vi "DFD Build MRate Filter from TF (Rational).vi"(6 "fs in [Hz]":dbl=1.0 format="%#_2g", 8 "error in (no error)":errorcluster, 10 "factor":T1, 11 "h(n)":dbl[](array[numeric])) -> (0 "error out":errorcluster, 3 "multirate filter out":T2={"mMRate_Structure"=enum."IIR", "mMRate_Mode"=0, "mMRate_Factor"=-1, "mMRate_FIRParams"={"mMRate_FIR_H"=[], "mMRate_FIR_IsNyquist?"=FALSE, "mMRate_FIR_IsSymmetric?"=FALSE}, "mMRate_CICParams"={"mMRate_CIC_#Stage"=0, "mMRate_CIC_Lag"=0, "mMRate_CIC_Type"=enum."Lowpass"}, "mMRate_Order"=0, "mMRate_Version"="2.0", "mMRate_Comments"="", "mMRate_RationalFactor"={"mMRate_L"=-1, "mMRate_M"=-1}, "mMRate_Fs"=1.0, "mMRate_Quantized?"=FALSE, "mMRate_QFilterGain"=1.0, "mMRate_CoefWl"=16, "mMRate_Scaling"={"mMRate_ScaleByPowerOf2?"=FALSE, "mMRate_ScaleType"=enum."No Norm"}, "mMRate_InputWl"=16, "mMRate_OutputWl"=16, "mMRate_OutputMode"=enum."Truncation", "mMRate_MultMode"=enum."Truncated", "mMRate_BitPruning"=FALSE, "mMRate_GainWl"=16, "mMRate_OutputFwl"=0, "mMRate_SumIwl"=0, "mMRate_InputIwl "=16, "mMRate_SumWl"=32, "mMRate_CoefIwl"=0} {"mMRate_SumWl" min=1 max=32 step=1; "mMRate_InputIwl" min=1 max=32 step=1; "mMRate_GainWl" min=1 max=32 step=1; "mMRate_OutputWl" min=1 max=32 step=1; "mMRate_InputWl" min=1 max=32 step=1; "mMRate_CoefWl" min=1 max=32 step=1; "mMRate_Mode" items=["Default"=-1, "No Rate Change"=0, "Interpolation"=1, "Decimation"=2, "Interpolated"=3, "Rational"=4]})   [LabVIEW 2017, in "NI_DigFilterLicensed.lvlib"]
doc: "Creates a multirate filter. You must manually select the polymorphic instance you want to use."
uses:
  <vilib>/addons/Digital Filter Design/NI_DigFilterLicensed.lvlib
  <vilib>/addons/Digital Filter Design/_Objects.llb/DFD Multirate Filter Obj.ctl
  <vilib>/addons/Digital Filter Design/_Objects.llb/DFD Multirate Mode.ctl
  <vilib>/addons/Digital Filter Design/_Objects.llb/DFD Coef Norm Type.ctl
  <vilib>/addons/Digital Filter Design/_Objects.llb/DFD Round-off Mode.ctl
  <vilib>/addons/Digital Filter Design/_Objects.llb/DFD FXP MRate Multiply Mode.ctl
  <vilib>/addons/Digital Filter Design/_Objects.llb/DFD Multirate Rational Factor.ctl
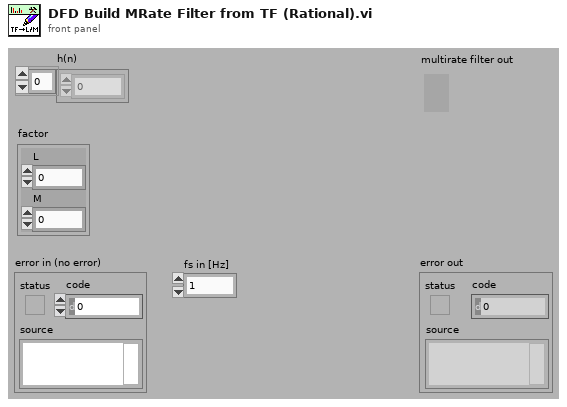
[diagram p1: front panel]
types:
  T1 = typedef "NI_DigFilterLicensed.lvlib/DFD Multirate Rational Factor.ctl" = cluster{"L":i32, "M":i32}
  T2 = typedef "NI_DigFilterLicensed.lvlib/DFD Multirate Filter Obj.ctl" = cluster{"mMRate_Structure":enum16{"CIC", "FIR", "IIR", "Lattice"}, "mMRate_Mode":T3, "mMRate_Factor":i32, "mMRate_FIRParams":cluster{"mMRate_FIR_H":dbl[], "mMRate_FIR_IsNyquist?":bool, "mMRate_FIR_IsSymmetric?":bool}, "mMRate_CICParams":cluster{"mMRate_CIC_#Stage":i32, "mMRate_CIC_Lag":i32, "mMRate_CIC_Type":enum16{"Lowpass", "Highpass"}}, "mMRate_Order":i32, "mMRate_Version":string, "mMRate_Comments":string, "mMRate_RationalFactor":cluster{"mMRate_L":i32, "mMRate_M":i32}, "mMRate_Fs":dbl, "mMRate_Quantized?":bool, "mMRate_QFilterGain":dbl, "mMRate_CoefWl":i16, "mMRate_Scaling":cluster{"mMRate_ScaleByPowerOf2?":bool, "mMRate_ScaleType":T4}, "mMRate_InputWl":i16, "mMRate_OutputWl":i16, "mMRate_OutputMode":T5, "mMRate_MultMode":T6, "mMRate_BitPruning":bool, "mMRate_GainWl":i16, "mMRate_OutputFwl":i16, "mMRate_SumIwl":i16, "mMRate_InputIwl ":i16, "mMRate_SumWl":i16, "mMRate_CoefIwl":i16}
  T3 = typedef "NI_DigFilterLicensed.lvlib/DFD Multirate Mode.ctl" = i16
  T4 = typedef "NI_DigFilterLicensed.lvlib/DFD Coef Norm Type.ctl" = enum16{"No Norm", "Time Domain 1-Norm", "Time Domain 2-Norm", "Time Domain Inf-Norm"}
  T5 = typedef "NI_DigFilterLicensed.lvlib/DFD Round-off Mode.ctl" = enum16{"Nearest", "Truncation"}
  T6 = typedef "NI_DigFilterLicensed.lvlib/DFD FXP MRate Multiply Mode.ctl" = enum16{"Truncated", "Full"}
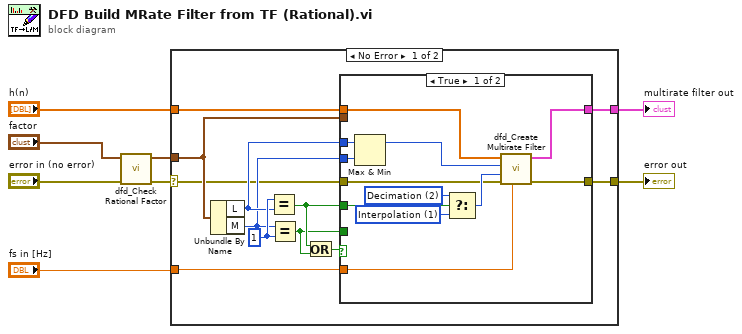
[diagram p0: block diagram]
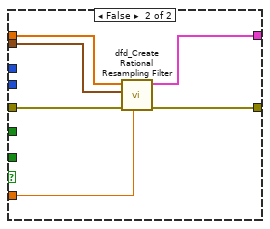
[diagram p2: hidden frame]
diagram:
  n1 = call <vilib>:"dfd_Check Rational Factor.vi"("error in (no error)"="error in (no error)", "rational factor in"="factor") -> ("error out"=w4:errorcluster, "rational factor out"=w6:T1)  [unwired: 8 out]
  n2 = case shown="No Error" w4 {
    selector: w4 -> [w11 w39]
    tunnel: "h(n)" -> [w19 _]
    tunnel: [w20 _] -> w8
    tunnel: w6 -> [w14 _]
    tunnel: [w10 w39] -> w3
    tunnel: "fs in [Hz]" -> [w9 _]
    frame No Error {
      w15 = 1 ("x")
      n3 = Unbundle By Name(w14) -> ("L"=w13:i32, "M"=w12:i32)
      n4 = Equal?(x=w15, y=w13) -> (x = y?=w18:bool)
      n5 = Equal?(x=w12, y=w15) -> (x = y?=w17:bool)
      n6 = Or(x=w18, y=w17) -> (x .or. y?=w16:bool)
      n7 = case shown="True" w16 {
        tunnel: [w27 w38] -> w20
        tunnel: w19 -> [w29 w36]
        tunnel: w14 -> [_ w37]
        tunnel: w18 -> [w32 _]
        tunnel: w17 -> [_ _]
        tunnel: w13 -> [w31 _]
        tunnel: w12 -> [w30 _]
        tunnel: w11 -> [w24 w35]
        tunnel: [w23 w34] -> w10
        tunnel: w9 -> [w21 w33]
        frame True {
          w25 = T3 1 items=["Default"=-1, "No Rate Change"=0, "Interpolation"=1, "Decimation"=2, "Interpolated"=3, "Rational"=4] ("mode")
          w22 = T3 2 items=["Default"=-1, "No Rate Change"=0, "Interpolation"=1, "Decimation"=2, "Interpolated"=3, "Rational"=4] ("mode")
          n8 = Max & Min(x=w31, y=w30) -> (max(x,y)=w26:i32)  [unwired: 1 out]
          n9 = Select(t=w22, s=w32, f=w25) -> (s? t:f=w28:T3)
          n10 = call <vilib>:"dfd_Create Multirate Filter.vi"("fs"=w21, "error in (no error)"=w24, "mode"=w28, "factor"=w26, "h (n)"=w29) -> ("error out"=w23:errorcluster, "multirate filter out"=w27:T2)  [unwired: 5 out]
        }
        frame False {
          n11 = call <vilib>:"dfd_Create Rational Resampling Filter.vi"("fs"=w33, "error in (no error)"=w35, "rational factor out"=w37, "validated numerator"=w36) -> ("error out"=w34:errorcluster, "multirate filter out"=w38:T2)  [unwired: 6 out]
        }
      }
    }
    frame Error {
    }
  }
  "error out" <- w3
  "multirate filter out" <- w8
